vi "Configure Tasks And Channels.vi"(11 "DAQmx Shortcuts":T1[](array[typedef])) -> (2 "Task Per Device":refnum<k21>[](array[refnum]), 3 "DAQmx Shortcuts Per Device":cluster{T1[]}[](array[cluster]))   [LabVIEW 2019, in "LINX.lvlib" / "LINX.lvclass"]
doc: "Map channels to devices, creating one task per device with those channels. Output is a jagged 2D array of devices & channels, where there could be 1-n channels per device."
uses:
  LINX.lvclass
  <resource>/objmgr/daqmx.rc
  LINX Shortcut.ctl
  <vilib>/DAQmx/configure/timing.llb/DAQmx Timing (Sample Clock).vi
  LINX Channel Type.ctl
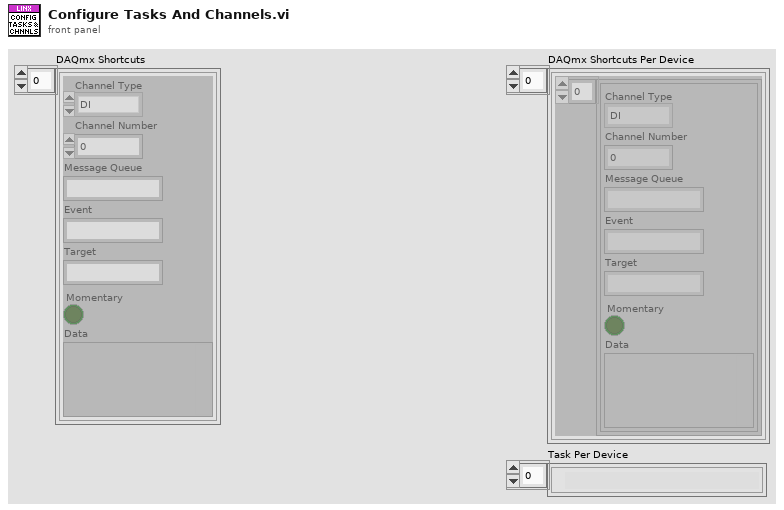
[diagram p1: front panel]
types:
  T1 = typedef "LINX.lvlib/LINX.lvclass/LINX Shortcut.ctl" = cluster{"Channel Type":T2, "Channel Number":u8, "Message Queue":string, "Event":string, "Target":string, "Momentary":bool, "Data":variant}
  T2 = typedef "LINX.lvlib/LINX.lvclass/LINX Channel Type.ctl" = enum16{"DI", "AI"}
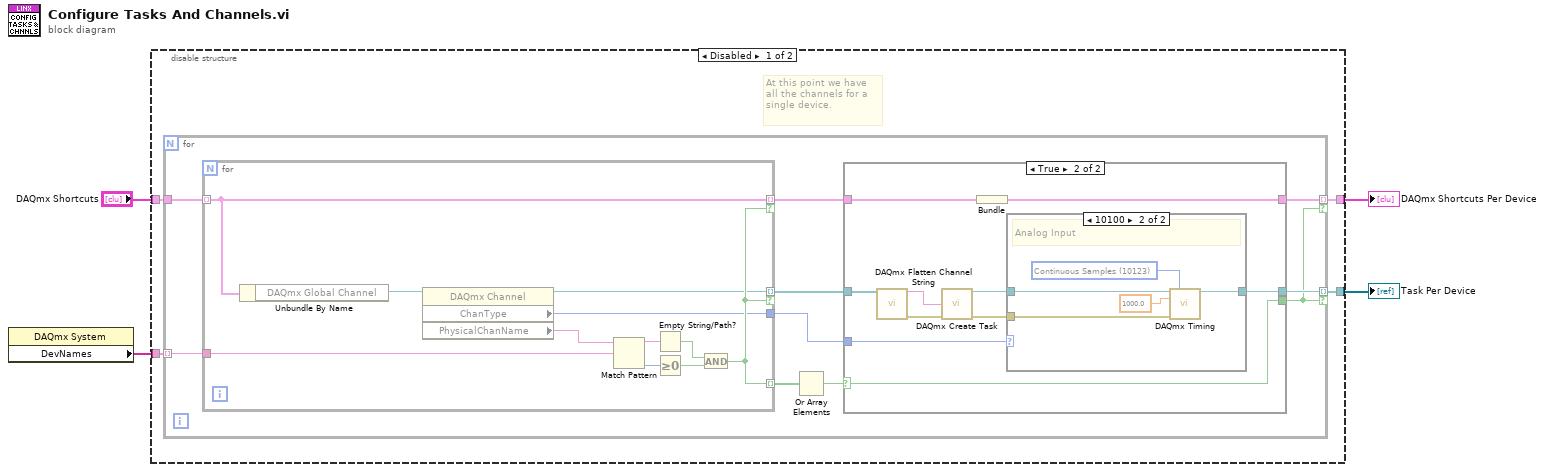
[diagram p0: block diagram]
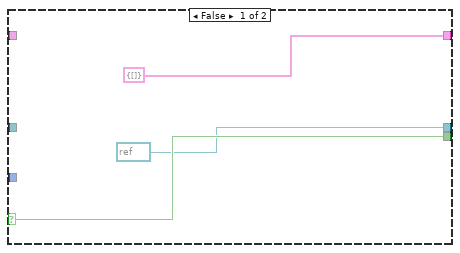
[diagram p2: hidden frame]
diagram:
  n1 = property class="DAQmx System"() -> ("DevNames"=w4:tag[])  [unwired: 2 in, 2 out]
  n2 = disable-structure shown="Disabled" {
    disable-tunnel: w4 -> [w8 _]
    disable-tunnel: "DAQmx Shortcuts" -> [w7 _]
    disable-tunnel: [w6 _] -> w2
    disable-tunnel: [w5 _] -> w1
    frame Disabled {
      # "At this point we have all the channels for a single device."
      n3 = for {
        tunnel: w8 -> [w18] mode=indexing
        tunnel: [w14] -> w5 mode=indexing if=w12
        tunnel: w7 -> [w13]
        tunnel: [w10] -> w6 mode=indexing if=w12
        n4 = for {
          tunnel: w18 -> [w48]
          tunnel: [w43] -> w17 mode=indexing
          tunnel: [w41] -> w15 mode=indexing if=w43
          tunnel: w13 -> [w40] mode=indexing
          tunnel: [w40] -> w11 mode=indexing if=w43
          tunnel: [w38] -> w9
          n5 = Unbundle By Name(w40) -> ("DAQmx Global Channel"=w39:refnum<k21>)
          n6 = property class="DAQmx Channel"(reference=w39) -> (reference out=w41:refnum<k21>, "ChanType"=w38:i32, "PhysicalChanName"=w42:tag)  [unwired: 1 in, 1 out]
          n7 = Match Pattern(string=w42, regular expression=w48) -> (before substring=w47:string, offset past match=w46:i32)  [unwired: 1 in, 2 out]
          n8 = Empty String/Path?(string/path=w47) -> (empty?=w45:bool)
          n9 = Greater Or Equal To 0?(x=w46) -> (x >= 0?=w44:bool)
          n10 = And(x=w45, y=w44) -> (x .and. y?=w43:bool)
        }
        n11 = Or Array Elements(Boolean array=w17) -> (logical OR=w16:bool)
        n12 = case shown="True" w16 {
          selector: w16 -> [w21 w26]
          tunnel: w15 -> [_ w25]
          tunnel: [refnum<k21> refnum ("task out") w27] -> w14
          tunnel: [w21 w26] -> w12
          tunnel: w11 -> [_ w24]
          tunnel: [cluster{T1[]} {[]} w23] -> w10
          tunnel: w9 -> [_ w22]
          frame False {
          }
          frame True {
            n13 = call <vilib>:"DAQmx Flatten Channel String.vi"("names in"=w25) -> ("names out"=w29:string, "error out"=w28:errorcluster)  [unwired: 13 in]
            n14 = call <vilib>:"DAQmx Create Task.vi"("global virtual channels"=w29, "error in"=w28) -> ("task out"=w31:refnum<k21>, "error out"=w30:errorcluster)  [unwired: 12 in]
            n15 = Bundle(w24) -> (w23:cluster{T1[]})  [unwired: 1 in]
            n16 = case shown="10100" w22 {
              tunnel: w31 -> [w32 w35]
              tunnel: w30 -> [_ w34]
              tunnel: [w32 w33] -> w27
              frame Default {
              }
              frame 10100 {
                w36 = 10123 items=["Finite Samples"=10178, "Continuous Samples"=10123, "Hardware Timed Single Point"=12522] ("sample mode")
                # "Analog Input"
                n17 = call-poly <vilib>:"DAQmx Timing.vi"("task/channels in"=w35, "sample mode"=w36, "rate"=1000.0, "error in"=w34) -> ("task out"=w33:refnum<k21>)  [unwired: 10 in, 1 out]
              }
            }
          }
        }
      }
    }
    frame Enabled {
    }
  }
  "DAQmx Shortcuts Per Device" <- w2
  "Task Per Device" <- w1
